vi "CLRWrapper_Test.vi"() -> ()   [LabVIEW 2020]
uses:
  Axis.lvclass
panel:
  in  "targetPosn":i32
  in  "Stop":bool=TRUE
  out "MoveDone":bool
  out "Waveform Chart":T1(graph)
  out "Error":bool
  out "Error Status Message":string
  out "scaledPosn":i64
  in  "ComPortHub":u64
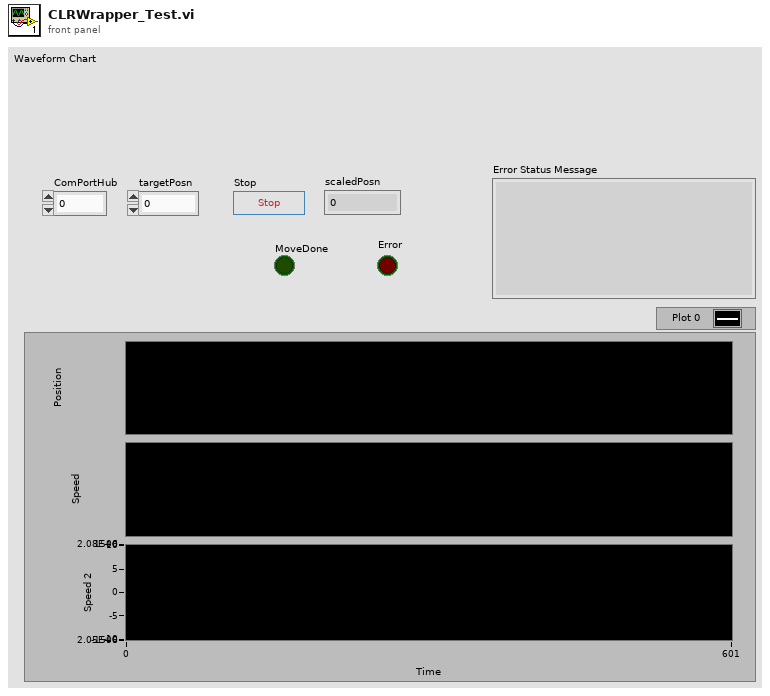
[diagram p1: front panel]
types:
  T1 = cluster{"scaledPosn":i64, "Velocity":dbl, "Torque":dbl}
  T2 = cluster{"scaledPosn":i64, "Velocity":dbl, "Torque":dbl}[]
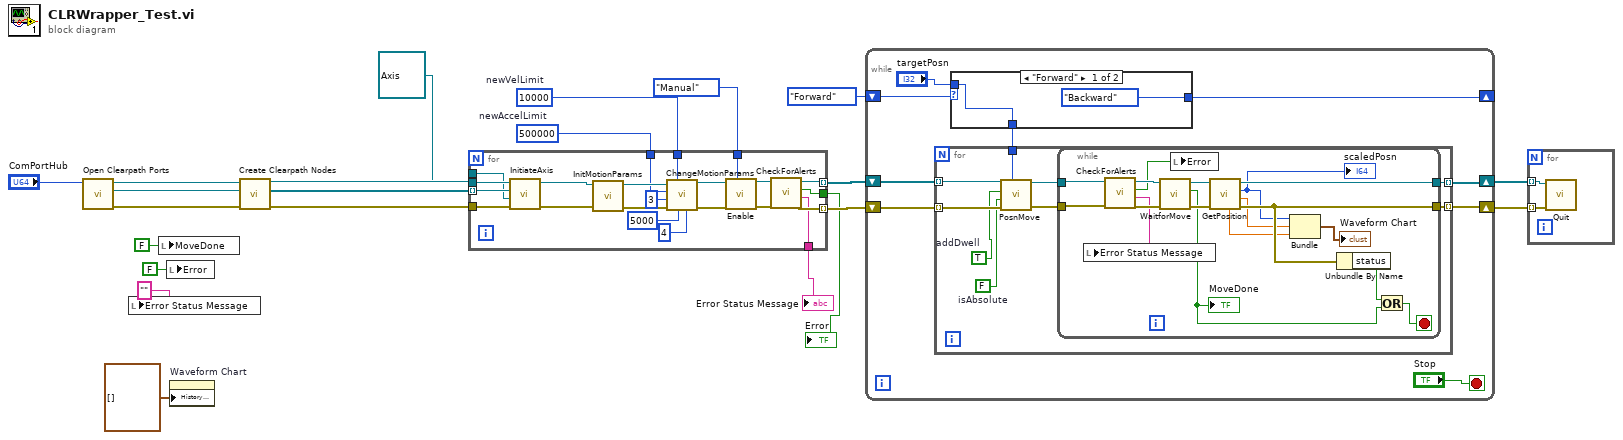
[diagram p0: block diagram]
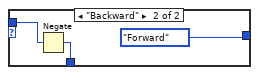
[diagram p2: hidden frame]
diagram:
  w10 = 500000  # newAccelLimit
  w11 = 10000  # newVelLimit
  n1 = call "Open Clearpath Ports.vi"("ComPortHub"="ComPortHub") -> ("error out"=w22:errorcluster, "ComHubPortOut"=w17:refnum<k24>, "m_SzsMgrOut"=w18:refnum<k24>)  [unwired: 8 in]
  n2 = local write "Error Status Message"("" ("ToString")) -> ()
  n3 = local write "MoveDone"(FALSE ("MoveDone")) -> ()
  n4 = local write "Error"(FALSE ("Error")) -> ()
  n5 = property on="Waveform Chart" class="WFChart (strict)"("History Data"=T2 []) -> ()  [unwired: 2 in, 2 out]
  n6 = call "Create Clearpath Nodes.vi"("error in (no error)"=w22, "ComHubPortIn"=w17, "m_SysMgrIn"=w18) -> ("error out"=w21:errorcluster, "NodeList"=w20:refnum<k24>[], "m_SysMgrOut"=w16:refnum<k24>)  [unwired: 4 in, 1 out]
  n7 = for {
    tunnel: refnum<class "Axis.lvclass"> refnum ("Axis.lvclass") -> [w44]
    tunnel: w21 -> [w43]
    tunnel: [w30] -> w9 mode=indexing
    tunnel: w20 -> [w42] mode=indexing
    tunnel: [w29] -> w8 mode=indexing
    tunnel: w16 -> [w41]
    tunnel: w11 -> [w34]
    tunnel: w10 -> [w33]
    tunnel: [w28] -> w7
    tunnel: [w27] -> w6
    tunnel: enum16{"Auto", "Manual"}."Manual" ("HomingMode") -> [w23]
    n8 = call "InitiateAxis.vi"("Axis in"=w44, "m_Node"=w42, "m_sysMgr"=w41, "error in (no error)"=w43) -> ("Axis out"=w39:refnum<class "Axis.lvclass">, "error out"=w40:errorcluster)  [unwired: 5 in]
    n9 = call "InitMotionParams.vi"("error in (no error)"=w40, "Axis in"=w39) -> ("error out"=w37:errorcluster, "Axis out"=w38:refnum<class "Axis.lvclass">)  [unwired: 8 in]
    n10 = call "ChangeMotionParams.vi"("newTrqGlobal"=4, "newTrackingLimit"=u32 5000, "newVelLimit"=w34, "error in (no error)"=w37, "newJrkLimit"=3, "newAccelLimit"=w33, "Axis in"=w38) -> ("error out"=w36:errorcluster, "Axis out"=w35:refnum<class "Axis.lvclass">)  [unwired: 3 in]
    n11 = call "Enable.vi"("HomingMode"=w23, "error in (no error)"=w36, "Axis in"=w35) -> ("error out"=w31:errorcluster, "Axis out"=w32:refnum<class "Axis.lvclass">)  [unwired: 7 in]
    n12 = call "CheckForAlerts.vi"("error in (no error)"=w31, "Axis in"=w32) -> ("error out"=w29:errorcluster, "ToString"=w28:string, "Boolean"=w27:bool, "Axis out"=w30:refnum<class "Axis.lvclass">)  [unwired: 6 in]
  }
  "Error Status Message" <- w7
  "Error" <- w6
  n13 = while {
    shift-right: [w51] -> w4
    shift-left: w9 -> [w53]
    shift-right: [w50] -> w3
    shift-left: w8 -> [w52]
    shift-right: [w48] -> _
    shift-left: enum16{"Forward", "Backward"}."Forward" -> [w49]
    stop <- "Stop" stop-if-true
    n14 = case shown="\"Forward\"" w49 {
      tunnel: [enum16{"Forward", "Backward"}."Backward" enum16{"Forward", "Backward"}."Forward"] -> w48
      tunnel: "targetPosn" -> [w54 w57]
      tunnel: [w54 w56] -> w46
      frame "Forward" {
      }
      frame "Backward" {
        n15 = Negate(x=w57) -> (-x=w56:i32)
      }
    }
    n16 = for {
      tunnel: [w65] -> w51 mode=indexing
      tunnel: w53 -> [w64] mode=indexing
      tunnel: w52 -> [w63] mode=indexing
      tunnel: [w62] -> w50 mode=indexing
      tunnel: w46 -> [w59]
      w61 = TRUE  # addDwell
      w60 = FALSE  # isAbsolute
      n17 = call "PosnMove.vi"("targetPosn"=w59, "error in (no error)"=w63, "isAbsolute"=w60, "addDwell"=w61, "Axis in"=w64) -> ("error out"=w67:errorcluster, "Axis out"=w66:refnum<class "Axis.lvclass">)  [unwired: 5 in]
      n18 = while {
        tunnel: w67 -> [w77]
        tunnel: w66 -> [w78]
        tunnel: [w82] -> w65
        tunnel: [w72] -> w62
        stop <- w79 stop-if-true
        n19 = call "CheckForAlerts.vi"("error in (no error)"=w77, "Axis in"=w78) -> ("error out"=w75:errorcluster, "ToString"=w74:string, "Boolean"=w73:bool, "Axis out"=w76:refnum<class "Axis.lvclass">)  [unwired: 6 in]
        n20 = local write "Error Status Message"(w74) -> ()
        n21 = call "WaitforMove.vi"("error in (no error)"=w75, "Axis in"=w76) -> ("error out"=w83:errorcluster, "MoveDone"=w80:bool, "Axis out"=w84:refnum<class "Axis.lvclass">)  [unwired: 7 in]
        "MoveDone" <- w80
        n22 = local write "Error"(w73) -> ()
        n23 = call "GetPosition.vi"("error in (no error)"=w83, "Axis in"=w84) -> ("error out"=w72:errorcluster, "Velocity"=w70:dbl, "scaledPosn"=w71:i64, "Axis out"=w82:refnum<class "Axis.lvclass">, "Torque"=w68:dbl)  [unwired: 5 in]
        "scaledPosn" <- w71
        n24 = Bundle("scaledPosn"=w71, "Velocity"=w70, "Torque"=w68) -> (→"Waveform Chart":T1)  [unwired: 1 in]
        n25 = Unbundle By Name(w72) -> ("status"=w81:bool)
        n26 = Or(x=w81, y=w80) -> (x .or. y?=w79:bool)
      }
    }
  }
  n27 = for {
    tunnel: w4 -> [w86] mode=indexing
    tunnel: w3 -> [w85] mode=indexing
    n28 = call-dynamic "Quit.vi"("error in (no error)"=w85, "Axis in"=w86) -> ()  [unwired: 8 in, 2 out]
  }
